vi "DATADYN.vi"(8 "errin":errorcluster, 10 "Limites":T2, 11 "3P4S":bool) -> (0 "errout":errorcluster caption="sortie d'erreur", 1 "CAN TIME out":bool, 2 "Out":T3, 3 "test OK?":bool, 4 "cluster de sortie":T1)   [LabVIEW 2020]
doc: "Test les modules via la carte CMOD"
uses:
  <userlib>/Alex_Peak_lib/PEAK_lib_ALEX.lvlib
  <userlib>/PCAN Basic/PCANBasic.lvlib
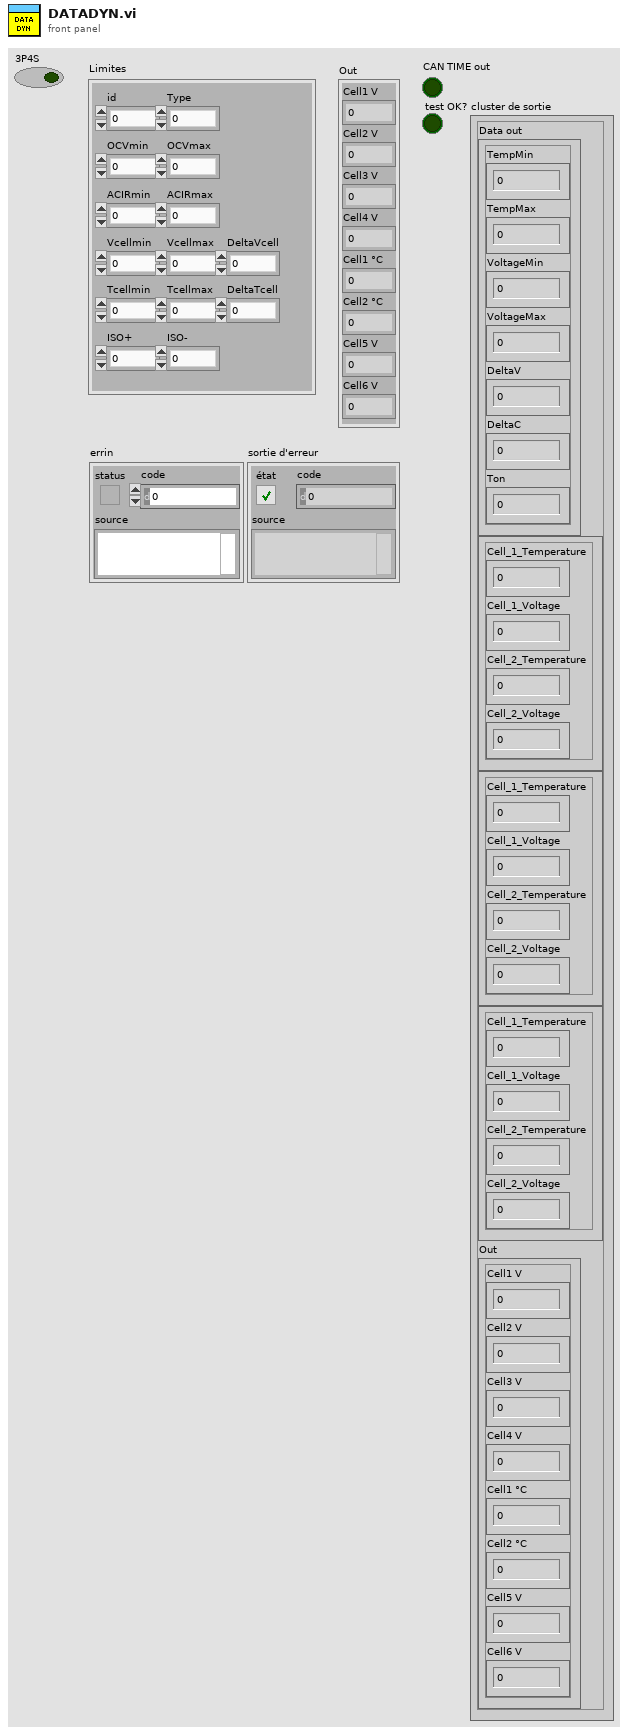
[diagram p1: front panel]
types:
  T1 = cluster{"Data out":cluster{"TempMin":sgl, "TempMax":sgl, "VoltageMin":sgl, "VoltageMax":sgl, "DeltaV":sgl, "DeltaC":sgl, "Ton":sgl}, "Cluster":cluster{"Cell_1_Temperature":sgl, "Cell_1_Voltage":sgl, "Cell_2_Temperature":sgl, "Cell_2_Voltage":sgl}, "Cluster":cluster{"Cell_1_Temperature":sgl, "Cell_1_Voltage":sgl, "Cell_2_Temperature":sgl, "Cell_2_Voltage":sgl}, "Cluster":cluster{"Cell_1_Temperature":sgl, "Cell_1_Voltage":sgl, "Cell_2_Temperature":sgl, "Cell_2_Voltage":sgl}, "Out":cluster{"Cell1 V":sgl, "Cell2 V":sgl, "Cell3 V":sgl, "Cell4 V":sgl, "Cell1 °C":sgl, "Cell2 °C":sgl, "Cell5 V":sgl, "Cell6 V":sgl}}
  T2 = cluster{"id":dbl, "Type":dbl, "OCVmin":dbl, "OCVmax":dbl, "ACIRmin":dbl, "ACIRmax":dbl, "Vcellmin":dbl, "Vcellmax":dbl, "DeltaVcell":dbl, "Tcellmin":dbl, "Tcellmax":dbl, "DeltaTcell":dbl, "ISO+":dbl, "ISO-":dbl}
  T3 = cluster{"Cell1 V":sgl, "Cell2 V":sgl, "Cell3 V":sgl, "Cell4 V":sgl, "Cell1 °C":sgl, "Cell2 °C":sgl, "Cell5 V":sgl, "Cell6 V":sgl}
  T4 = cluster{"TempMin":sgl, "TempMax":sgl, "VoltageMin":sgl, "VoltageMax":sgl, "DeltaV":sgl, "DeltaC":sgl, "Ton":sgl}
  T5 = typedef "PCANBasic.lvlib/Channel.ctl" = enum16{"PCAN_NONEBUS", "not used1", "not used2", "not used3", "not used4", "not used5", "not used6", "not used7", "not used8", "not used9", "not used10", "not used11", "not used12", "not used13", "not used14", "not used15", "not used16", "not used17", "not used18", "not used19", "not used20", "not used21", "not used22", "not used23", "not used24", "not used25", "not used26", "not used27", "not used28", "not used29", "not used30", "not used31", "not used32", "PCAN_ISABUS1", "PCAN_ISABUS2", "PCAN_ISABUS3", "PCAN_ISABUS4", "PCAN_ISABUS5", "PCAN_ISABUS6", "PCAN_ISABUS7", "PCAN_ISABUS8", "not used41", "not used42", "not used43", "not used44", "not used45", "not used46", "not used47", "not used48", "PCAN_DNGBUS1", "not used50", "not used51", "not used52", "not used53", "not used54", "not used55", "not used56", "not used57", "not used58", "not used59", "not used60", "not used61", "not used62", "not used63", "not used64", "PCAN_PCIBUS1", "PCAN_PCIBUS2", "PCAN_PCIBUS3", "PCAN_PCIBUS4", "PCAN_PCIBUS5", "PCAN_PCIBUS6", "PCAN_PCIBUS7", "PCAN_PCIBUS8", "not used73", "not used74", "not used75", "not used76", "not used77", "not used78", "not used79", "not used80", "PCAN_USBBUS1", "PCAN_USBBUS2", "PCAN_USBBUS3", "PCAN_USBBUS4", "PCAN_USBBUS5", "PCAN_USBBUS6", "PCAN_USBBUS7", "PCAN_USBBUS8", "Not used89", "Not used90", "Not used91", "Not used92", "Not used93", "Not used94", "Not used95", "Not used96", "PCAN_PCCBUS1", "PCAN_PCCBUS2"}
  T6 = cluster{"Cell_1_Temperature":sgl, "Cell_1_Voltage":sgl, "Cell_2_Temperature":sgl, "Cell_2_Voltage":sgl}
  T7 = cluster{"ID":u32, "MSGTYPE":u8, "LEN":u8, "DATA[0]":u8, "DATA[1]":u8, "DATA[2]":u8, "DATA[3]":u8, "DATA[4]":u8, "DATA[5]":u8, "DATA[6]":u8, "DATA[7]":u8}
  T8 = cluster{"Cell1 V":string, "Cell2 V":string, "Cell3 V":string, "Cell4 V":string, "Cell1 °C":string, "Cell2 °C":string, "Cell5 V":string, "Cell6 V":string}
  T9 = cluster{"Data out":cluster{"TempMin":sgl, "TempMax":sgl, "VoltageMin":sgl, "VoltageMax":sgl, "DeltaV":sgl, "DeltaC":sgl, "Ton":sgl}, cluster{"Cell_1_Temperature":sgl, "Cell_1_Voltage":sgl, "Cell_2_Temperature":sgl, "Cell_2_Voltage":sgl}, cluster{"Cell_1_Temperature":sgl, "Cell_1_Voltage":sgl, "Cell_2_Temperature":sgl, "Cell_2_Voltage":sgl}, cluster{"Cell_1_Temperature":sgl, "Cell_1_Voltage":sgl, "Cell_2_Temperature":sgl, "Cell_2_Voltage":sgl}, "Out":cluster{"Cell1 V":sgl, "Cell2 V":sgl, "Cell3 V":sgl, "Cell4 V":sgl, "Cell1 °C":sgl, "Cell2 °C":sgl, "Cell5 V":sgl, "Cell6 V":sgl}}
  T10 = cluster{"millis":u32, "millis_overflow":u16, "micros":u16}
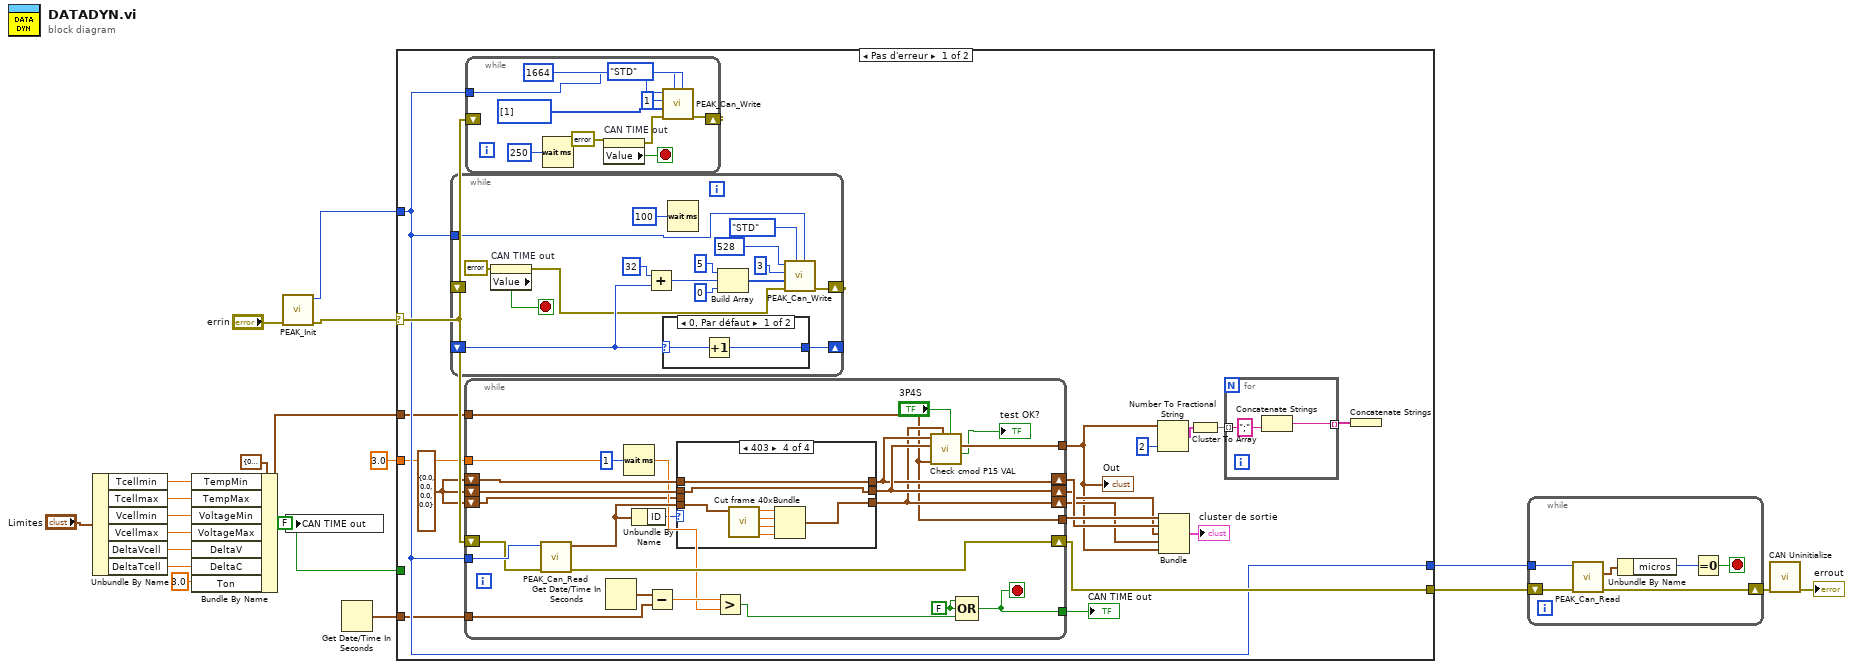
[diagram p0: block diagram]
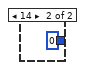
[diagram p2: hidden frame]
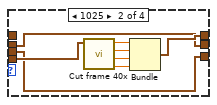
[diagram p4: hidden frame]
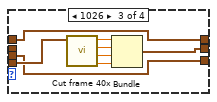
[diagram p5: hidden frame]
diagram:
  w18 = FALSE ("Booléen")
  n1 = Unbundle By Name("Limites") -> ("Tcellmin"=w10:dbl, "Tcellmax"=w9:dbl, "Vcellmin"=w8:dbl, "Vcellmax"=w7:dbl, "DeltaVcell"=w6:dbl, "DeltaTcell"=w5:dbl)
  n2 = Bundle By Name(cluster=T4 {"TempMin"=0.0, "TempMax"=0.0, "VoltageMin"=0.0, "VoltageMax"=0.0, "DeltaV"=0.0, "DeltaC"=0.0, "Ton"=0.0} ("Data out"), "TempMin"=w10, "TempMax"=w9, "VoltageMin"=w8, "VoltageMax"=w7, "DeltaV"=w6, "DeltaC"=w5, "Ton"=sgl 3.0) -> (w2:T4)
  n3 = call <userlib>:"PEAK_Init.vi"("errin"="errin") -> ("errout"=w16:errorcluster, "Channel out"=w17:T5)  [unwired: 9 in]
  n4 = local write "CAN TIME out"(w18) -> ()
  n5 = Get Date/Time In Seconds() -> (seconds since 1Jan1904=w19:timestamp)
  n6 = case shown="Pas d'erreur" w16 {
    selector: w16 -> [w38 w122]
    tunnel: w17 -> [w36 w121]
    tunnel: [w37 w122] -> w15
    tunnel: [w36 w121] -> w14
    tunnel: w19 -> [w34 _]
    tunnel: w2 -> [w33 _]
    tunnel: 3.0 ("Timeout") -> [w32 _]
    tunnel: w18 -> [_ _]
    frame No Error {
      w27 = T6 {"Cell_1_Temperature"=0.0, "Cell_1_Voltage"=0.0, "Cell_2_Temperature"=0.0, "Cell_2_Voltage"=0.0}
      n7 = while {
        tunnel: w36 -> [w52]
        shift-right: [w67] -> _
        shift-left: _ -> [w66]
        shift-right: [w65] -> _
        shift-left: w38 -> [_]
        stop <- w63 stop-if-true
        n8 = property on="CAN TIME out" class="Bool (strict)"(error in=errorcluster {"status"=FALSE, "code"=0, "source"=""} ("entrée d'erreur (pas d'erreur)")) -> (error out=w64:errorcluster, "Value"=w63:bool)  [unwired: 1 in, 1 out]
        n9 = Add(x=u8 32, y=w66) -> (x+y=w58:i32)
        n10 = case shown="0, Par défaut" w66 {
          selector: w66 -> [w69 _]
          tunnel: [w68 0] -> w67
          frame 0, Default {
            n11 = Increment(x=w69) -> (x+1=w68:i32)
          }
          frame 14 {
          }
        }
        n12 = Wait (ms)(milliseconds to wait=u32 100 ("attente (ms)")) -> ()  [unwired: 1 out]
        n13 = Build Array(u8 5 ("élément"), w58, u8 0 ("élément")) -> (w57:i32[])
        n14 = call <userlib>:"PEAK_Can_Write.vi"("CAN Handle"=w52, "MSG type"=enum8{"STD", "RTR", "XTD", "XTD RTR", "STATUS"}."STD", "errin"=w64, "CAN Data"=w57, "DLC (8)"=u8 3, "Identifier"=u32 528) -> ("errout"=w65:errorcluster)  [unwired: 5 in]
      }
      n15 = while {
        shift-right: [w87] -> w37
        shift-left: w38 -> [w91]
        shift-right: [w85] -> w25
        shift-left: w27 -> [w89]
        shift-right: [w86] -> w24
        shift-left: w27 -> [w88]
        tunnel: w36 -> [w92]
        tunnel: [w84] -> w22
        tunnel: [w83] -> w35
        tunnel: w34 -> [w79]
        tunnel: w33 -> [w71]
        tunnel: w32 -> [w78]
        shift-right: [w74] -> w23
        shift-left: w27 -> [w77]
        tunnel: [w71] -> w26
        stop <- w83 stop-if-true
        w75 = FALSE ("valeur")
        n16 = call <userlib>:"PEAK_Can_Read.vi"("errin"=w91, "Channel out"=w92) -> ("errout"=w87:errorcluster, "MessageBuffer out"=w90:T7)  [unwired: 7 in, 1 out]
        n17 = Get Date/Time In Seconds() -> (seconds since 1Jan1904=w80:timestamp)
        n18 = Wait (ms)(milliseconds to wait=u32 1 ("attente (ms)")) -> ()  [unwired: 1 out]
        n19 = Unbundle By Name(w90) -> ("ID"=w76:u32)
        n20 = Subtract(x=w80, y=w79) -> (x-y=w81:dbl)
        n21 = case shown="403" w76 {
          tunnel: w90 -> [_ w99 w107 w116]
          tunnel: [w96 w100 w106 w114] -> w85
          tunnel: [w95 w98 w108 w113] -> w86
          tunnel: w89 -> [w96 _ w106 w114]
          tunnel: w88 -> [w95 w98 _ w113]
          tunnel: [w94 w97 w105 w115] -> w74
          tunnel: w77 -> [w94 w97 w105 _]
          frame 0, Default {
          }
          frame 1025 {
            n22 = call "Cut frame 40x.vi"("MessageBuffer out"=w99) -> ("Cell_2_Voltage"=w101:sgl, "Cell_2_Temperature"=w102:sgl, "Cell_1_Voltage"=w103:sgl, "Cell_1_Temperature"=w104:sgl)  [unwired: 7 in]
            n23 = Bundle("Cell_1_Temperature"=w104, "Cell_1_Voltage"=w103, "Cell_2_Temperature"=w102, "Cell_2_Voltage"=w101) -> (w100:T6)  [unwired: 1 in]
          }
          frame 1026 {
            n24 = call "Cut frame 40x.vi"("MessageBuffer out"=w107) -> ("Cell_2_Voltage"=w109:sgl, "Cell_2_Temperature"=w110:sgl, "Cell_1_Voltage"=w111:sgl, "Cell_1_Temperature"=w112:sgl)  [unwired: 7 in]
            n25 = Bundle("Cell_1_Temperature"=w112, "Cell_1_Voltage"=w111, "Cell_2_Temperature"=w110, "Cell_2_Voltage"=w109) -> (w108:T6)  [unwired: 1 in]
          }
          frame 1027 {
            n26 = call "Cut frame 40x.vi"("MessageBuffer out"=w116) -> ("Cell_2_Voltage"=w117:sgl, "Cell_2_Temperature"=w118:sgl, "Cell_1_Voltage"=w119:sgl, "Cell_1_Temperature"=w120:sgl)  [unwired: 7 in]
            n27 = Bundle("Cell_1_Temperature"=w120, "Cell_1_Voltage"=w119, "Cell_2_Temperature"=w118, "Cell_2_Voltage"=w117) -> (w115:T6)  [unwired: 1 in]
          }
        }
        n28 = Greater?(x=w81, y=w78) -> (0:w82:bool)
        n29 = call "Check cmod P15 VAL.vi"("3P4S"="3P4S", "Cell 5 et 6"=w74, "Limites"=w71, "Cell 3 et 4"=w86, "Cell 1 et 2"=w85) -> ("ok global"=→"test OK?":bool, "Out"=w84:T3)  [unwired: 2 in, 3 out]
        n30 = Compound Arithmetic op=OR(w75, w75, w82) -> (w83:bool)
      }
      "CAN TIME out" <- w35
      "Out" <- w22
      n31 = while {
        tunnel: w36 -> [w44]
        shift-right: [w48] -> _
        shift-left: w38 -> [_]
        stop <- w51 stop-if-true
        n32 = Wait (ms)(milliseconds to wait=u32 250 ("attente (ms)")) -> ()  [unwired: 1 out]
        n33 = property on="CAN TIME out" class="Bool (strict)"(error in=errorcluster {"status"=FALSE, "code"=0, "source"=""} ("entrée d'erreur (pas d'erreur)")) -> (error out=w47:errorcluster, "Value"=w51:bool)  [unwired: 1 in, 1 out]
        n34 = call <userlib>:"PEAK_Can_Write.vi"("CAN Handle"=w44, "MSG type"=enum8{"STD", "RTR", "XTD", "XTD RTR", "STATUS"}."STD", "errin"=w47, "CAN Data"=u8[] [1], "DLC (8)"=u8 1, "Identifier"=u32 1664) -> ("errout"=w48:errorcluster)  [unwired: 5 in]
      }
      n35 = Number To Fractional String ("Nombre en chaîne fractionnaire")(number=w22, precision (6)=i16 2 ("précision (6)")) -> (F-format string=w30:T8)  [unwired: 2 in]
      n36 = Bundle("Data out"=w26, w25, w24, w23, "Out"=w22) -> (→"cluster de sortie":T9)  [unwired: 1 in]
      n37 = Cluster To Array(cluster=w30) -> (array=w29:string[])
      n38 = for {
        tunnel: w29 -> [w40] mode=indexing
        tunnel: [w39] -> w28 mode=indexing
        n39 = Concatenate Strings(w40, ";" ("chaîne")) -> (w39:string)
      }
      n40 = Concatenate Strings(w28) -> ()  [unwired: 1 out]
    }
    frame Error {
    }
  }
  n41 = while {
    tunnel: w14 -> [w127]
    shift-right: [w126] -> w13
    shift-left: w15 -> [w128]
    stop <- w124 stop-if-true
    n42 = call <userlib>:"PEAK_Can_Read.vi"("errin"=w128, "Channel out"=w127) -> ("errout"=w126:errorcluster, "TimestampBuffer out 2"=w123:T10)  [unwired: 7 in, 1 out]
    n43 = Unbundle By Name(w123) -> ("micros"=w125:u16)
    n44 = Equal To 0?(x=w125) -> (x = 0?=w124:bool)
  }
  n45 = call <userlib>:"CAN Uninitialize.vi"("error in (no error)"=w13) -> ("error out"=→"errout":errorcluster)  [unwired: 8 in, 2 out]
